vi "Configure.vi"(0 "session in":T6[](array[typedef]) {"rx baseband session"."3630 session"."Address Space" items=["VXI/VME A16"=1, "VXI/VME A24"=2, "VXI/VME A32"=3, "VXI/VME A64"=4, "PXI Memory Allocations"=9, "PXI Configuration"=10, "PXI BAR0"=11, "PXI BAR1"=12, "PXI BAR2"=13, "PXI BAR3"=14, "PXI BAR4"=15, "PXI BAR5"=16]; "tx baseband session"."3610 session"."Address Space" items=["VXI/VME A16"=1, "VXI/VME A24"=2, "VXI/VME A32"=3, "VXI/VME A64"=4, "PXI Memory Allocations"=9, "PXI Configuration"=10, "PXI BAR0"=11, "PXI BAR1"=12, "PXI BAR2"=13, "PXI BAR3"=14, "PXI BAR4"=15, "PXI BAR5"=16]}, 7 "device configuration [channel]":T3[](array[typedef])=[{"port select"=enum."Loopback", "Rx hardware configuration"={"gain (dB)"=15.0, "frequency (Hz)"=12000000000.0, "mmWave adapter"="None", "adapter active port"=""}, "Tx hardware configuration"={"gain (dB)"=-15.0, "frequency (Hz)"=12000000000.0, "mmWave adapter"="None", "adapter active port"=""}}] {"Tx hardware configuration"."frequency (Hz)" format="%#_6p"; "Rx hardware configuration"."frequency (Hz)" format="%#_6p"}, 11 "error in":errorcluster, 12 "LO sources":T2={"RX/LO1 src"="Internal", "TX/LO1 src"="Internal", "LO2 src"="Internal"}, 13 "LO Export":T1) -> (4 "session out":T6[](array[typedef]) {"rx baseband session"."3630 session"."Address Space" items=["VXI/VME A16"=1, "VXI/VME A24"=2, "VXI/VME A32"=3, "VXI/VME A64"=4, "PXI Memory Allocations"=9, "PXI Configuration"=10, "PXI BAR0"=11, "PXI BAR1"=12, "PXI BAR2"=13, "PXI BAR3"=14, "PXI BAR4"=15, "PXI BAR5"=16]; "tx baseband session"."3610 session"."Address Space" items=["VXI/VME A16"=1, "VXI/VME A24"=2, "VXI/VME A32"=3, "VXI/VME A64"=4, "PXI Memory Allocations"=9, "PXI Configuration"=10, "PXI BAR0"=11, "PXI BAR1"=12, "PXI BAR2"=13, "PXI BAR3"=14, "PXI BAR4"=15, "PXI BAR5"=16]}, 8 "coerced device configuration [channel]":T3[](array[typedef])=[{"port select"=enum."Loopback", "Rx hardware configuration"={"gain (dB)"=15.0, "frequency (Hz)"=12000000000.0, "mmWave adapter"="None", "adapter active port"=""}, "Tx hardware configuration"={"gain (dB)"=-15.0, "frequency (Hz)"=12000000000.0, "mmWave adapter"="None", "adapter active port"=""}}] {"Tx hardware configuration"."frequency (Hz)" format="%#_6p"; "Rx hardware configuration"."frequency (Hz)" format="%#_6p"}, 15 "error out":errorcluster)   [LabVIEW 2019, in "mmWave HW Control.lvlib"]
uses:
  mmWave HW Control.lvlib
  Low-level/TypeDefs/Front End Configuration.ctl
  Low-level/TypeDefs/Channel Configuration.ctl
  <instrlib>/niMmWave/ni3620/Config/v1/Host/Public/Typedefs/mmWave Port.ctl
  Low-level/TypeDefs/Session.ctl
  <instrlib>/niMmWave/ni3620/Config/v1/Host/Public/High-Level/niMmWave Session.ctl
  <instrlib>/_niInstr/Register Bus/v0/Host/Public/Register Bus Session.ctl
  <instrlib>/_niInstr/Register Bus/v0/Host/Private/Session Data.ctl
  <instrlib>/niMmWave/ni3620/Config/v1/Host/Public/Typedefs/Board Information.ctl
  <instrlib>/niMmWave/ni3620/Config/v1/Host/Public/Typedefs/Hardware Revision.ctl
  <instrlib>/niMmWave/ni3620/Config/v1/Host/Public/Typedefs/Gain Mapping.ctl
  <instrlib>/niMmWave/ni3620/Config/v1/Host/Public/Typedefs/Correction Data.ctl
  <instrlib>/niMmWave/ni3620/Config/v1/Host/Public/Typedefs/Opera Characterization.ctl
  <instrlib>/niMmWave/ni3620/Config/v1/Host/Public/Corrections/Typedefs/Opera Characterization Main Header.ctl
  <instrlib>/niMmWave/ni3620/Config/v1/Host/Public/Corrections/Typedefs/Opera IF Board Information.ctl
  <instrlib>/niMmWave/ni3620/Config/v1/Host/Public/Corrections/Typedefs/Opera Characterization Instance Header.ctl
  <instrlib>/niMmWave/ni3620/Config/v1/Host/Public/Corrections/Typedefs/Opera Characterization Device Data Header.ctl
  <instrlib>/niMmWave/ni3620/Config/v1/Host/Public/Corrections/Typedefs/Opera LO Characterization Data Header.ctl
  <instrlib>/niMmWave/ni3620/Config/v1/Host/Public/Corrections/Typedefs/Opera IF Board Characterization Data Header.ctl
  <instrlib>/niMmWave/ni3620/Config/v1/Host/Public/Corrections/Typedefs/Opera Characterization Device Data.ctl
  <instrlib>/niMmWave/ni3620/Config/v1/Host/Public/Corrections/Typedefs/Opera LO2 Board Characterization Data.ctl
  <instrlib>/niMmWave/ni3620/Config/v1/Host/Public/Corrections/Typedefs/Opera LO Characterization Data.ctl
  <instrlib>/niMmWave/ni3620/Config/v1/Host/Public/Corrections/Typedefs/Opera IF Board Characterization Data.ctl
  <instrlib>/niMmWave/ni3620/Config/v1/Host/Public/Corrections/Typedefs/Opera IQ Impairment Data.ctl
  <instrlib>/niMmWave/ni3620/Config/v1/Host/Public/Typedefs/mmWave Adapter Session Data.ctl
  <instrlib>/niMmWave/ni3620/Config/v1/Host/Public/Typedefs/mmWave Adapter Data.ctl
  <instrlib>/niMmWave/ni3620/Config/v1/Host/Public/Typedefs/mmWave Adapter 2.ctl
  <instrlib>/niMmWave/ni3620/Config/v1/Shared/Typedefs/Subsystem ID.ctl
  <instrlib>/niMmWave/ni3620/Config/v1/Host/Public/Typedefs/mmWave Adapter Channel Information.ctl
  <instrlib>/niMmWave/ni3620/Config/v1/Host/Public/Typedefs/Temperature Coefficients.ctl
  <instrlib>/niMmWave/ni3620/Config/v1/Host/Public/Typedefs/mmWave Characterization.ctl
  <instrlib>/niMmWave/ni3620/Config/v1/Host/Public/Corrections/Typedefs/mmWave Characterization Main Header.ctl
  <instrlib>/niMmWave/ni3620/Config/v1/Host/Public/Corrections/Typedefs/mmWave Characterization Instance Header.ctl
  <instrlib>/niMmWave/ni3620/Config/v1/Host/Public/Typedefs/Session Cache.ctl
  <instrlib>/niMmWave/ni3620/Config/v1/Host/Public/Typedefs/LO2 settings cache.ctl
  <instrlib>/niMmWave/ni3620/Config/v1/Host/Public/Typedefs/LO2 source.ctl
  <instrlib>/niMmWave/ni3620/Config/v1/Host/Public/Typedefs/Desired and Coerced.ctl
  <instrlib>/niMmWave/ni3620/Config/v1/Host/Public/Typedefs/Export cache.ctl
  <instrlib>/niMmWave/ni3620/Config/v1/Host/Public/Typedefs/Path cache.ctl
  <instrlib>/niMmWave/ni3620/Config/v1/Host/Public/Typedefs/Daughterboard Type.ctl
  <instrlib>/niMmWave/ni3620/Config/v1/Host/Public/Typedefs/LO1 settings cache.ctl
  <instrlib>/niMmWave/ni3620/Config/v1/Host/Public/Typedefs/LO1 Source.ctl
  <instrlib>/niMmWave/ni3620/Config/v1/Host/Public/Typedefs/mmWave export cache.ctl
  <instrlib>/niMmWave/ni3620/Config/v1/Host/Private/Board/LO2/LO2 Board Configuration Cache.ctl
  <instrlib>/niMmWave/ni3620/Config/v1/Host/Public/Typedefs/reference clock routing settings.ctl
  <instrlib>/niMmWave/ni3620/Config/v1/Host/Public/Typedefs/LO2 routing settings.ctl
  <instrlib>/niMmWave/ni3620/Config/v1/Host/Private/Board/LO1/LO1 Board Configuration Cache.ctl
  <instrlib>/niMmWave/ni3620/Config/v1/Host/Public/Typedefs/LO1 source settings.ctl
  <instrlib>/niMmWave/ni3620/Config/v1/Host/Public/Typedefs/LO1 export settings.ctl
  <instrlib>/niMmWave/ni3620/Config/v1/Host/Public/Typedefs/LO1 mmWave settings.ctl
  Low-level/TypeDefs/Tx Baseband Session.ctl
  <instrlib>/niMmWave/ni3610 and ni3630/controls/public/Main Settings.ctl
  <vilib>/Instr/_visa.llb/VISA Register Access Address Space.ctl
  <instrlib>/niMmWave/ni3610 and ni3630/controls/public/Register Adresses.ctl
  <instrlib>/niMmWave/ni3610 and ni3630/controls/public/Base Card Type.ctl
  <instrlib>/niMmWave/ni3610 and ni3630/controls/private/IQ Card Revision.ctl
  <instrlib>/niMmWave/ni3610 and ni3630/controls/public/Board Capability.ctl
  Low-level/TypeDefs/Blank FPGA Reference.ctl
  Low-level/TypeDefs/Rx Baseband Session.ctl
  Low-level/TypeDefs/Hardware Configuration.ctl
  Low-level/TypeDefs/Direction.ctl
  Low-level/TypeDefs/Gain Ranging.ctl
  Low-level/TypeDefs/PXI Trigger Bus Info.ctl
  LO sources.ctl
  LO export.ctl
  <instrlib>/niMmWave/ni3620/Config/v1/Host/Public/Typedefs/Rx IF signal source.ctl
  <instrlib>/niMmWave/ni3620/Config/v1/Host/Public/Typedefs/Tx IF signal destination.ctl
  <instrlib>/niMmWave/ni3620/Config/v1/Host/niMmWave Config v1 Host.lvlib
  <instrlib>/niMmWave/ni3610 and ni3630/ni3610_and_ni3630_Driver_Lib.lvlib
  <instrlib>/_niInstr/Register Bus/v0/Host/niInstr Register Bus v0 Host.lvlib
  <instrlib>/niMmWave/ni3620/Config/v1/Shared/niMmWave Config v1 Shared.lvlib
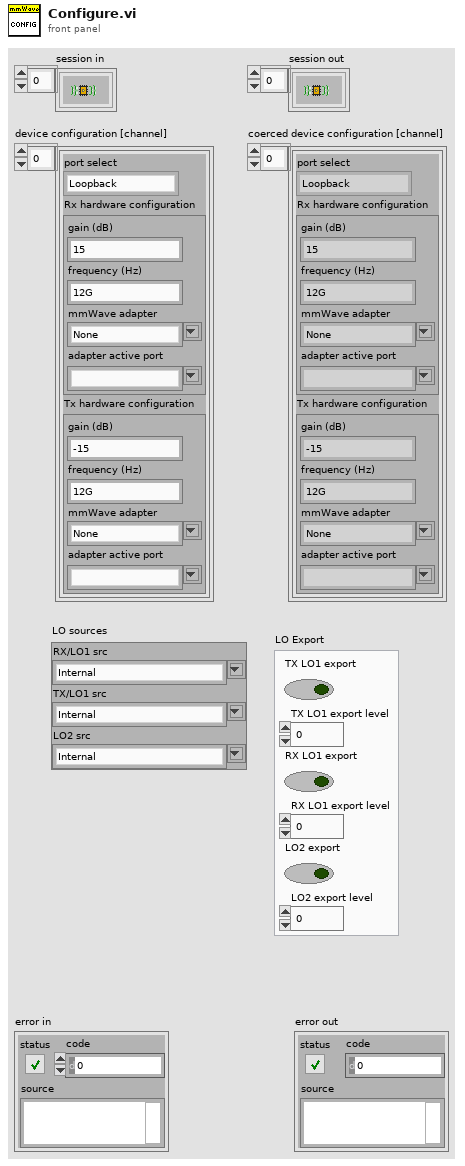
[diagram p1: front panel]
types:
  T1 = typedef "mmWave HW Control.lvlib/LO export.ctl" = cluster{"TX LO1 export":bool, "TX LO1 export level":dbl, "RX LO1 export":bool, "RX LO1 export level":dbl, "LO2 export":bool, "LO2 export level":dbl}
  T2 = typedef "mmWave HW Control.lvlib/LO sources.ctl" = cluster{"RX/LO1 src":string, "TX/LO1 src":string, "LO2 src":string}
  T3 = typedef "Front End Configuration.ctl" = cluster{"port select":enum16{"IF Port", "Loopback", "Sync Port"}, "Rx hardware configuration":T4, "Tx hardware configuration":T4}
  T4 = typedef "Channel Configuration.ctl" = cluster{"gain (dB)":dbl, "frequency (Hz)":dbl, "mmWave adapter":string, "adapter active port":T5}
  T5 = typedef "niMmWave Config v1 Host.lvlib/mmWave Port.ctl" = string
  T6 = typedef "Session.ctl" = cluster{"3620 session":refnum<queue>, "tx baseband session":T7, "rx baseband session":T15, "tx gain (dB)":dbl, "rx gain (dB)":dbl, "hardware configuration":T16, "gain ranging":T18[], "pxi trigger bus information":T19}
  T7 = typedef "Tx Baseband Session.ctl" = cluster{"3610 session":T8, "7902 reference":T14}
  T8 = typedef "ni3610_and_ni3630_Driver_Lib.lvlib/Main Settings.ctl" = cluster{"VISA resource name":refnum<visa-resource-name>, "Address Space":T9, "window_offset":u32, "register_addresses":T10, "required_MM_fpga_version":cluster{"signature":u32, "hardware":u32, "current revision":u32, "oldest revision":u32}, "CPLD Oldest Compat Version ":cluster{"hardware":u32, "CPLD firmware":u32}, "MM_FPGA_image_location":string, "is_init":bool, "card_type":T11, "DacLmkConfigFileName":string, "AdcLmkConfigFileName":string, "AdcConfigFileName":string, "DacConfigFileName_RevA":string, "DacConfigFileName_RevB":string, "Mulde hardware revision":u8, "bypass DAC PLL\n":bool, "IQ Card Revision":T12, "board capability":T13}
  T9 = typedef "VISA Register Access Address Space.ctl" = u16
  T10 = typedef "ni3610_and_ni3630_Driver_Lib.lvlib/Register Adresses.ctl" = cluster{"MM based Registers":cluster{"Revision":u32, "OldestCompatRev":u32, "signature":u32, "scratch":u32, "LedControl":u32, "BoardHwRev":u32, "BoardControl":u32, "ThermalStatus":u32, "BasebandStatus":u32, "BasebandControl":u32, "BasebandAuxSetup":u32, "BasebandAuxStatus":u32, "LmkSyncOutSetup":u32, " AdcSyncOutSetup":u32, " InjSyncOutSetup":u32, " PxiTrig0OutSetup":u32, " PxiTrig1OutSetup":u32, " PxiTrig2OutSetup":u32, " PxiTrig3OutSetup":u32, " PxiTrig4OutSetup":u32, " PxiTrig5OutSetup":u32, " PxiTrig6OutSetup":u32, " PxiTrig7OutSetup":u32}, "CPLD based Registers":cluster{"SlaveSignature":u32, "SlaveRevision":u32, "SlaveOldestCompatRev":u32, "SlaveScratch":u32, "SlaveSetup":u32, "SlaveStatus":u32, "IDacReg_offset":u32, "LMKRegGrp0_offset":u32, "QDacReg_offset":u32, "BrdTempSensorVal":u32, "TempSensorPowerDown":u32, "GPIOReg_offset":u32, "IAdcReg_offset":u32, "QAdcReg_offset":u32, "LMKRegGrp1_offset":u32, "QadcTempSensorVal":u32, "IadcTempSensorVal":u32, "RevisionReg":u32, "VcxoReg":u32, "CpldStatusReg":u32, "PowerReg":u32, "VBiasEnReg":u32, "ExtRefOeReg":u32, "QdacCtrlReg":u32, "QdacStatusReg":u32, "IdacCtrlReg":u32, "IdacStatusReg":u32, "QdacJtagIn":u32, "QdacJtagOut":u32, "IdacJtagIn":u32, "IdacJtagOut":u32, "IqDcSetupReg":u32, "QadcStatusReg":u32, "IadcStatusReg":u32, "BrdSetupReg":u32, "IqDcRevisionReg":u32, "PllStatusReg":u32, "EndpointScratchReg":u32, "AdcSyncCfgReg":u32, "IqCardOpampReg":u32}, "CPLD Register Offset":u32, "MM  Register Offset":u32, " PxiTrig0OutSetup":u32}
  T11 = typedef "ni3610_and_ni3630_Driver_Lib.lvlib/Base Card Type.ctl" = enum16{"unspecified", "ADC", "DAC"}
  T12 = typedef "ni3610_and_ni3630_Driver_Lib.lvlib/IQ Card Revision.ctl" = enum16{"RevA", "RevB", "RevC", "RevD"}
  T13 = typedef "ni3610_and_ni3630_Driver_Lib.lvlib/Board Capability.ctl" = cluster{"baseband sync":enum16{"no baseband sync", "baseband sync"}}
  T14 = typedef "Blank FPGA Reference.ctl" = refnum<k20>
  T15 = typedef "Rx Baseband Session.ctl" = cluster{"3630 session":T8, "7902 reference":T14}
  T16 = typedef "Hardware Configuration.ctl" = cluster{"direction":T17, "baseband only":bool}
  T17 = typedef "Direction.ctl" = enum16{"Transceiver", "Receiver", "Transmitter"}
  T18 = typedef "Gain Ranging.ctl" = cluster{"gain ranging active scope":string, "gain ranging stream session":refnum<k20>}
  T19 = typedef "PXI Trigger Bus Info.ctl" = cluster{"chassis resource name":refnum<visa-resource-name>, "7902R (TX)":i16, "3610 (TX)":i16, "3620 (IF)":i16, "3630 (RX)":i16, "7902R (RX)":i16}
  T20 = typedef "niMmWave Config v1 Host.lvlib/Tx IF signal destination.ctl" = enum16{"IF Output", "IF Loopback", "Cal Output", "Disabled"}
  T21 = typedef "niMmWave Config v1 Host.lvlib/Rx IF signal source.ctl" = enum16{"IF Input", "IF Loopback", "External Cal Input", "Internal Cal Input"}
  T22 = typedef "niMmWave Config v1 Host.lvlib/Opera IQ Impairment Data.ctl" = cluster{"Gain Imbalance (linear)":dbl, "Phase Offset (radians)":dbl, "Offset ":cdb}
  T23 = typedef "niMmWave Config v1 Host.lvlib/IQ Inversion.ctl" = cluster{"invert i":bool, "invert q":bool}
  T24 = typedef "niMmWave Config v1 Host.lvlib/niMmWave Session.ctl" = cluster{"register bus ":T25, "board information":T26, "IF gain tables":cluster{"Gain Table":T28[]}[], "IF channel correction data":T29[], "ni3620 characterization data":T30, "mmWave adapter session data":T41, "session cache":T50, "lo2 board configuration cache":T60, "lo1 rx board configuration cache":T63, "lo1 tx board configuration cache":T63}
  T25 = typedef "niInstr Register Bus v0 Host.lvlib/Register Bus Session.ctl" = refnum<queue>
  T26 = typedef "niMmWave Config v1 Host.lvlib/Board Information.ctl" = cluster{"product code":u16, "hardware revision":T27, "serial number":u64}
  T27 = typedef "niMmWave Config v1 Host.lvlib/Hardware Revision.ctl" = enum16{"Unknown", "A", "B", "C", "D", "E", "F", "G", "H", "I", "J"}
  T28 = typedef "niMmWave Config v1 Host.lvlib/Gain Mapping.ctl" = cluster{"Gain":dbl, "Gain Settings":variant[]}
  T29 = typedef "niMmWave Config v1 Host.lvlib/Correction Data.ctl" = cluster{"Frequencies (Hz)":dbl[], "Nominal Gain Values (dB)":dbl[], "Measured Gain Values (dB)":dbl[][]}
  T30 = typedef "niMmWave Config v1 Host.lvlib/Opera Characterization.ctl" = cluster{"Characterization Data Valid?":bool, "ni3620 characterization main header":T31, "ni3620 characterization instance header":T33, "ni3620 characterization device data header":T34, "ni3620 characterization device data":T37}
  T31 = typedef "niMmWave Config v1 Host.lvlib/Opera Characterization Main Header.ctl" = cluster{"Header Checksum":u32, "Product Code":u16, "Module Serial Number":u64, "Hardware Current Version":u16, "Hardware Oldest Compatible Version":u16, "EEPROM Map Current Version":u16, "EEPROM Map Oldest Compatible Version":u16, "User Password":string, "Factory Characterization Header Address":u32, "User Characterization Header Address":u32, "Recommended Correction Interval (months)":u16, "Mighty Mouse Hardware Current Version":u16, "Mighty Mouse Serial Number":u64, "LO2 Board Hardware Current Version":u16, "LO2 Board Serial Number":u64, "Number of IF Boards":u8, "IF Boards":T32[], "Future Growth":u16}
  T32 = typedef "niMmWave Config v1 Host.lvlib/Opera IF Board Information.ctl" = cluster{"IF Board ID":u16, "IF Board Hardware Current Version":u16, "IF Board Serial Number":u64}
  T33 = typedef "niMmWave Config v1 Host.lvlib/Opera Characterization Instance Header.ctl" = cluster{"Header Checksum":u32, "Characterization Date":timestamp, "Characterization Temperature (C)":dbl, "Miscellaneous Information":string, "Device Characterization Header Address":u32, "Future Growth":u16}
  T34 = typedef "niMmWave Config v1 Host.lvlib/Opera Characterization Device Data Header.ctl" = cluster{"Header Checksum":u32, "Number of LO2 Export Paths":u8, "LO2 Export Paths":T35[], "Number of IF Boards":u8, "IF Boards":T36[], "Characterization Data Address":u32, "Future Growth":u16}
  T35 = typedef "niMmWave Config v1 Host.lvlib/Opera LO Characterization Data Header.ctl" = cluster{"LO Path Number of Frequencies":u16, "LO Path Number of Gain Values":u16}
  T36 = typedef "niMmWave Config v1 Host.lvlib/Opera IF Board Characterization Data Header.ctl" = cluster{"Number of LO1 Export Paths":u8, "LO1 Export Paths":T35[], "IF Path Number of Gain Frequencies":u16, "IF Path Number of Gain Stages":u16, "IF Path Gain Stages Number of Gain Values":u16[], "IF Path Number of IQ Impairment Frequencies":u16}
  T37 = typedef "niMmWave Config v1 Host.lvlib/Opera Characterization Device Data.ctl" = cluster{"LO2 Board Characterization Data":T38, "IF Board Characterization Data":T40[]}
  T38 = typedef "niMmWave Config v1 Host.lvlib/Opera LO2 Board Characterization Data.ctl" = cluster{"Data Checksum":u32, "TXCO Reference DAC Value":u16, "LO2 Export Paths":T39[]}
  T39 = typedef "niMmWave Config v1 Host.lvlib/Opera LO Characterization Data.ctl" = cluster{"Frequencies":dbl[], "Gain Values":dbl[], "Measured Gain / Power Values":dbl[][]}
  T40 = typedef "niMmWave Config v1 Host.lvlib/Opera IF Board Characterization Data.ctl" = cluster{"Data Checksum":u32, "LO1 Export Paths":T39[], "IF Path Gain Frequencies":dbl[], "IF Path Gain Stages Gain Values":cluster{"Gain Values":dbl[]}[], "Measured Maximum Gain (dB)":dbl[], "IF Path Gain Stages Measured Gain Values (dB)":cluster{"Measured Gain Values (dB)":dbl[][]}[], "IF Path IQ Impairment Frequencies":dbl[], "Measured IQ Impairments":T22[]}
  T41 = typedef "niMmWave Config v1 Host.lvlib/mmWave Adapter Session Data.ctl" = cluster{"mmWave0 chain size":u8, "mmWave1 chain size ":u8, "mmWave adapters":T42[]}
  T42 = typedef "niMmWave Config v1 Host.lvlib/mmWave Adapter Data.ctl" = cluster{"scope":string, "mmWave Adapter type":T43, "board information":T26, "subsystem":T44, "serial address":u8, "channels":T45[], "channel gain tables":cluster{"Gain Table":T28[]}[], "channel correction data":T29[], "channel temperature coefficients":T46[], "characterization data":T47, "board configuration cache":variant}
  T43 = typedef "niMmWave Config v1 Host.lvlib/mmWave Adapter 2.ctl" = enum16{"None", "NI 3647 71-76 GHz", "NI 3657 71-76 GHz", "NI 5580 55-68 GHz", "NI 5580 55-68 GHz Prototype Deck", "NI 3602 27.5-29.5 GHz", "NI 3642 27.5-29.5 GHz", "NI 3652 27.5-29.5 GHz", "NI 3603 37.0-43.5 GHz", "NI 3643 37.0-43.5 GHz", "NI 3653 37.0-43.5 GHz", "NI 3602 24.25-33.40 GHz", "NI 3642 24.25-33.40 GHz", "NI 3652 24.25-33.40 GHz"}
  T44 = typedef "niMmWave Config v1 Shared.lvlib/Subsystem ID.ctl" = enum8{"Identification", "Board Config", "Rx LO1", "Tx LO1", "LO2", "mmWave0", "mmWave1", "Rx LO1 Core", "Tx LO1 Core", "LO2 Core", "mmWave0 Core", "mmWave1 Core", "Gain Ranging", "mmWave mapping"}
  T45 = typedef "niMmWave Config v1 Host.lvlib/mmWave Adapter Channel Information.ctl" = cluster{"channel":string, "supported ports":string[], "active port":string}
  T46 = typedef "niMmWave Config v1 Host.lvlib/Temperature Coefficients.ctl" = cluster{"frequencies (Hz)":dbl[], "gains (dB)":dbl[], "temp coefficients [gain][freq]":dbl[][]}
  T47 = typedef "niMmWave Config v1 Host.lvlib/mmWave Characterization.ctl" = cluster{"Characterization Data Valid?":bool, "mmWave Characterization Main Header":T48, "mmWave Characterization Instance Header":T49, "mmWave Characterization Device Data Header":variant, "mmWave Characterization Device Data":variant}
  T48 = typedef "niMmWave Config v1 Host.lvlib/mmWave Characterization Main Header.ctl" = cluster{"Header Checksum":u32, "Product Code":u16, "Serial Number":u64, "Hardware Current Version":u16, "Hardware Oldest Compatible Version":u16, "EEPROM Map Current Version":u16, "EEPROM Map Oldest Compatible Version":u16, "Hardware Capabilities":u8, "User Password":string, "Factory Characterization Header Address":u32, "User Characterization Header Address":u32, "Recommended Correction Interval (months)":u16, "Future Growth":u16}
  T49 = typedef "niMmWave Config v1 Host.lvlib/mmWave Characterization Instance Header.ctl" = cluster{"Header Checksum":u32, "Characterization Date":timestamp, "Characterization Temperature (C)":dbl, "Miscellaneous Information":string, "Device Characterization Header Address":u32, "Future Growth":u16}
  T50 = typedef "niMmWave Config v1 Host.lvlib/Session Cache.ctl" = cluster{"Gain Corrections Enabled":bool, "LO2 Settings":T51, "TxRx Path Settings":T55[], "LO Corrections Enabled":bool}
  T51 = typedef "niMmWave Config v1 Host.lvlib/LO2 settings cache.ctl" = cluster{"Source":T52, "Frequency":T53, "Export Settings":T54}
  T52 = typedef "niMmWave Config v1 Host.lvlib/LO2 source.ctl" = enum16{"Internal", "LO2_IN"}
  T53 = typedef "niMmWave Config v1 Host.lvlib/Desired and Coerced.ctl" = cluster{"Desired":dbl, "Coerced":dbl}
  T54 = typedef "niMmWave Config v1 Host.lvlib/Export cache.ctl" = cluster{"Export Enabled":bool, "Path Gain":T53}
  T55 = typedef "niMmWave Config v1 Host.lvlib/Path cache.ctl" = cluster{"Daughterboard":T56, "current mmWave Adapter":T43, "current mmWave adapter index":i32, "Channel Enabled":bool, "Gain":T53, "Frequency":T53, "LO1":T57, "IF Route":variant}
  T56 = typedef "niMmWave Config v1 Host.lvlib/Daughterboard Type.ctl" = enum16{"3620 RX", "3620 TX"}
  T57 = typedef "niMmWave Config v1 Host.lvlib/LO1 settings cache.ctl" = cluster{"Source":T58, "Frequency":T53, "LO1 mmWave":T59, "LO1 Export":T54}
  T58 = typedef "niMmWave Config v1 Host.lvlib/LO1 Source.ctl" = enum16{"Internal", "LO1_IN"}
  T59 = typedef "niMmWave Config v1 Host.lvlib/mmWave export cache.ctl" = cluster{"Export Settings":T54, "AGC Enabled":bool, "Doubler Enabled":bool}
  T60 = typedef "niMmWave Config v1 Host.lvlib/LO2 Board Configuration Cache.ctl" = cluster{"reference clock routing settings":T61, "LO2 routing settings":T62}
  T61 = typedef "niMmWave Config v1 Host.lvlib/reference clock routing settings.ctl" = cluster{"reference clock source":enum16{"PXI_Clk10", "Ref In"}, "export reference clock ":bool}
  T62 = typedef "niMmWave Config v1 Host.lvlib/LO2 routing settings.ctl" = cluster{"LO2 Source":T52, "export LO2":bool, "LO2 output attenuation":fxp<+,7,5>}
  T63 = typedef "niMmWave Config v1 Host.lvlib/LO1 Board Configuration Cache.ctl" = cluster{"LO1 source routing settings":T64, "LO1 export routing settings":T65, "LO1 mmWave routing settings":T66}
  T64 = typedef "niMmWave Config v1 Host.lvlib/LO1 source settings.ctl" = cluster{"LO1 source":T58, "LO1 source attenuation":fxp<+,7,5>}
  T65 = typedef "niMmWave Config v1 Host.lvlib/LO1 export settings.ctl" = cluster{"export LO1":bool, "LO1 export attenuation":fxp<+,7,5>}
  T66 = typedef "niMmWave Config v1 Host.lvlib/LO1 mmWave settings.ctl" = cluster{"LO1 mmWave route":enum16{"Chop Cal", "Doubler", "Bypass"}, "LO1 mmWave attenuation":fxp<+,5,5>}
  T67 = typedef "ni3610_and_ni3630_Driver_Lib.lvlib/Baseband IQ Characterization Device Data.ctl" = cluster{"Checksum":u32, "Channel Delay":dbl, "Imbalance":cluster{"Gain Imbalance":dbl, "Phase Imbalance":dbl}, "DC Offset":cluster{"I DC Offset":dbl, "Q DC Offset":dbl}}
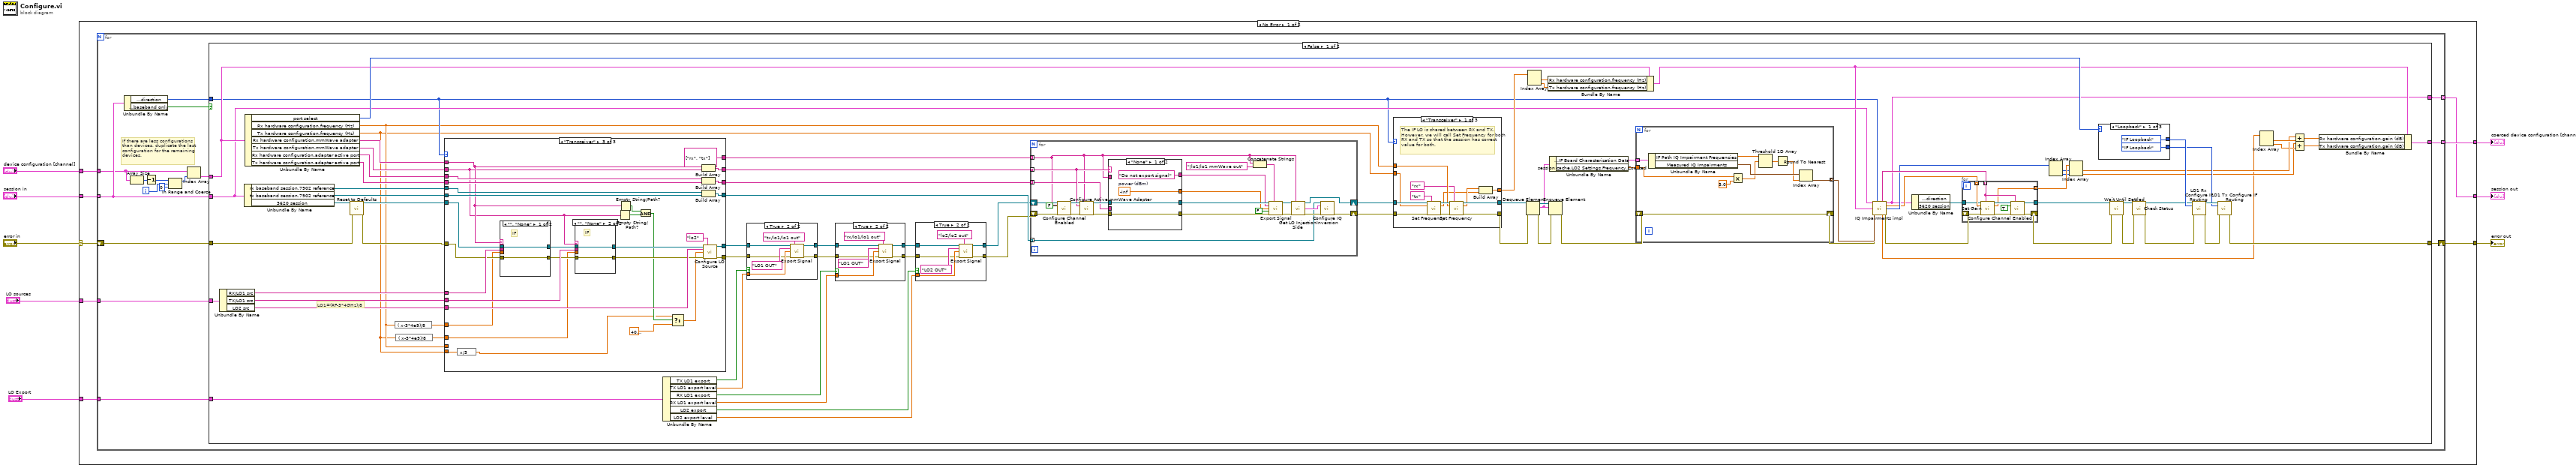
[diagram p0: block diagram]
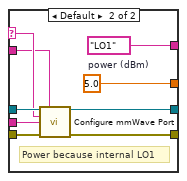
[diagram p5: hidden frame]
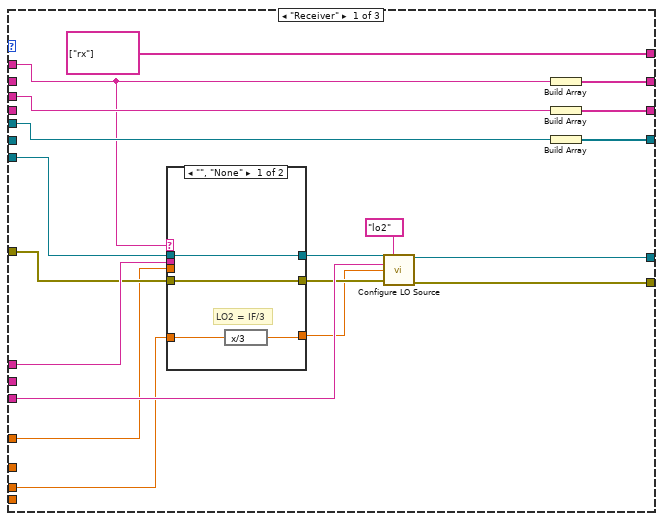
[diagram p6: hidden frame]
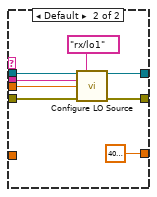
[diagram p7: hidden frame]
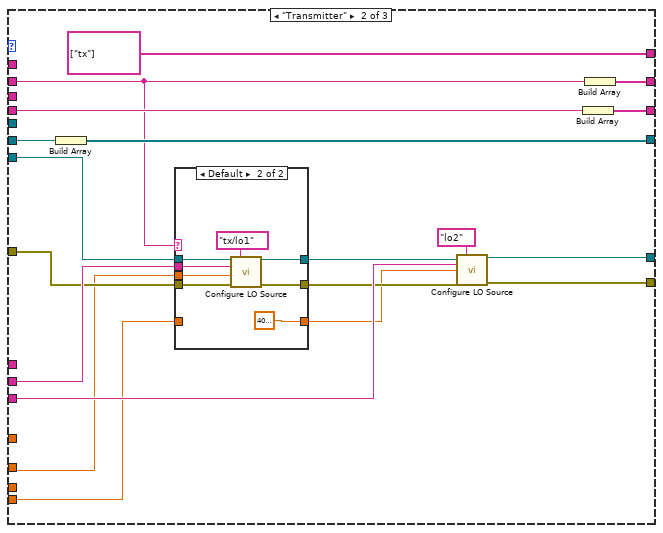
[diagram p8: hidden frame]
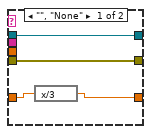
[diagram p9: hidden frame]
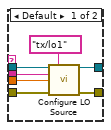
[diagram p10: hidden frame]
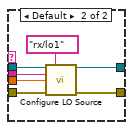
[diagram p11: hidden frame]
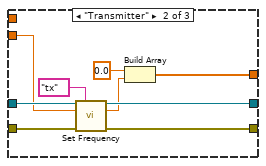
[diagram p12: hidden frame]
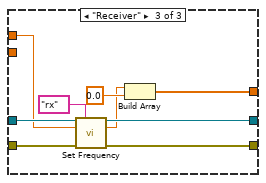
[diagram p13: hidden frame]
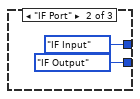
[diagram p14: hidden frame]
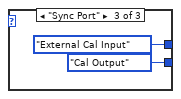
[diagram p15: hidden frame]
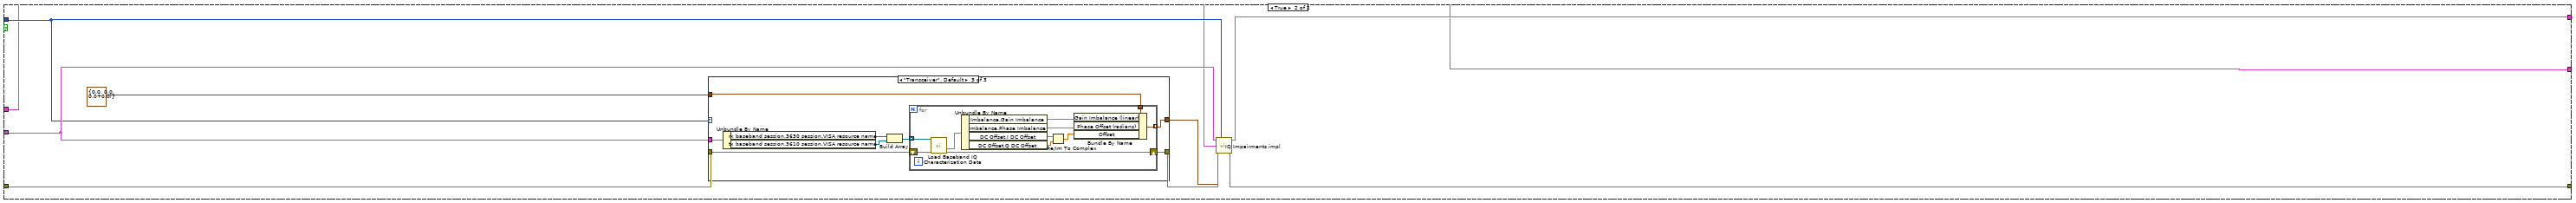
[diagram p16: hidden frame]
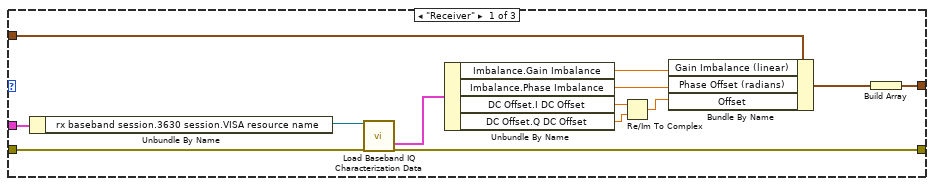
[diagram p17: hidden frame]
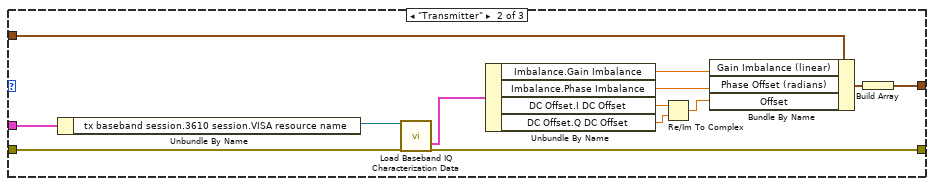
[diagram p18: hidden frame]
diagram:
  n1 = case shown="No Error" "error in" {
    selector: "error in" -> [w16 w405]
    tunnel: "device configuration [channel]" -> [w11 _]
    tunnel: "session in" -> [w12 w404]
    tunnel: [w15 w405] -> w7
    tunnel: [w14 _] -> w6
    tunnel: [w13 w404] -> w5
    tunnel: "LO sources" -> [w10 _]
    tunnel: "LO Export" -> [w9 _]
    frame No Error {
      n2 = for {
        shift-right: [w31] -> w15
        shift-left: w16 -> [w32]
        tunnel: w11 -> [w20]
        tunnel: [w30] -> w14 mode=indexing
        tunnel: w12 -> [w21] mode=indexing
        tunnel: [w29] -> w13 mode=indexing
        tunnel: w10 -> [w18]
        tunnel: w9 -> [w17]
        i -> [w22]
        # "If there are less configurations than devices, duplicate the last configuration for the remaining devices."
        n3 = Unbundle By Name(w21) -> ("hardware configuration.direction"=w28:T17, "hardware configuration.baseband only"=w27:bool)
        n4 = Array Size(array=w20) -> (size(s)=w25:i32)
        n5 = Decrement(x=w25) -> (x-1=w24:i32)
        n6 = In Range and Coerce(upper limit=w24, x=w22, lower limit=0) -> (coerced(x)=w23:i32)  [unwired: 1 out]
        n7 = Index Array(array=w20, index=w23) -> (element=w19:T3)
        n8 = case shown="False" w27 {
          tunnel: w19 -> [w86 w350]
          tunnel: w32 -> [w69 w358]
          tunnel: w21 -> [w68 w352]
          tunnel: [w93 w354] -> w31
          tunnel: w28 -> [w58 w351]
          tunnel: [w105 w350] -> w30
          tunnel: [w60 w353] -> w29
          tunnel: w18 -> [w57 _]
          tunnel: w17 -> [w49 _]
          frame False {
            # "LO1=(RF-3*4GHz)/8"
            n9 = Unbundle By Name(w57) -> ("RX/LO1 src"=w54:string, "TX/LO1 src"=w53:string, "LO2 src"=w52:string)
            n10 = Unbundle By Name(w68) -> ("rx baseband session.7902 reference"=w76:T14, "tx baseband session.7902 reference"=w75:T14, "3620 session"=w70:refnum<queue>)
            n11 = Unbundle By Name(w86) -> ("port select"=w109:enum16{"IF Port", "Loopback", "Sync Port"}, "Rx hardware configuration.frequency (Hz)"=w34:dbl, "Tx hardware configuration.frequency (Hz)"=w33:dbl, "Rx hardware configuration.mmWave adapter"=w80:string, "Tx hardware configuration.mmWave adapter"=w79:string, "Rx hardware configuration.adapter active port"=w73:T5, "Tx hardware configuration.adapter active port"=w71:T5)
            n12 = call <instrlib>:"Reset to Defaults.vi"("session in"=w70, "error in"=w69) -> ("session out"=w56:refnum<queue>, "error out"=w55:errorcluster)  [unwired: 12 in]
            n13 = expression code="( x-3*4e9)/8"(w34) -> (w51:dbl)
            n14 = expression code="( x-3*4e9)/8"(w33) -> (w50:dbl)
            n15 = case shown="\"Transceiver\"" w58 {
              tunnel: [string[] ["rx"] ("Array") string[] ["tx"] ("Array") string[] ["rx", "tx"] ("Array")] -> w82
              tunnel: [w199 w230 w273] -> w81
              tunnel: w80 -> [w184 _ w250]
              tunnel: w79 -> [_ w215 w248]
              tunnel: w76 -> [w198 _ w272]
              tunnel: w75 -> [_ w229 w270]
              tunnel: [w197 w228 w271] -> w74
              tunnel: w73 -> [w195 _ w269]
              tunnel: [w196 w227 w267] -> w72
              tunnel: w71 -> [_ w226 w268]
              tunnel: w56 -> [w194 w223 w263]
              tunnel: w55 -> [w188 w219 w258]
              tunnel: [w191 w222 w262] -> w47
              tunnel: w54 -> [w190 _ w261]
              tunnel: w53 -> [_ w220 w260]
              tunnel: w52 -> [w189 w221 w259]
              tunnel: [w186 w217 w255] -> w46
              tunnel: w51 -> [w185 _ w254]
              tunnel: w50 -> [_ w216 w253]
              tunnel: w34 -> [w182 _ _]
              tunnel: w33 -> [_ w213 w249]
              frame "Receiver" {
                n16 = case shown="\"\", \"None\"" w184 {
                  tunnel: w194 -> [w204 w212]
                  tunnel: [w204 w210] -> w193
                  tunnel: w190 -> [_ w209]
                  tunnel: w188 -> [w203 w208]
                  tunnel: [w203 w207] -> w187
                  tunnel: w185 -> [_ w206]
                  tunnel: [w201 4000000000.0 ("frequency (Hz)")] -> w183
                  tunnel: w182 -> [w202 _]
                  frame "", "None" {
                    # "LO2 = IF/3"
                    n17 = expression code="x/3"(w202) -> (w201:dbl)
                  }
                  frame Default {
                    n18 = call <instrlib>:"Configure LO Source.vi"("session in"=w212, "scope"="rx/lo1", "LO source"=w209, "frequency (Hz)"=w206, "error in"=w208) -> ("session out"=w210:refnum<queue>, "error out"=w207:errorcluster)  [unwired: 9 in]
                  }
                }
                n19 = call <instrlib>:"Configure LO Source.vi"("session in"=w193, "scope"="lo2", "LO source"=w189, "frequency (Hz)"=w183, "error in"=w187) -> ("session out"=w191:refnum<queue>, "error out"=w186:errorcluster)  [unwired: 9 in]
                n20 = Build Array(w184) -> (w199:string[])
                n21 = Build Array(w195) -> (w196:T5[])
                n22 = Build Array(w198) -> (w197:T14[])
              }
              frame "Transmitter" {
                n23 = Build Array(w229) -> (w228:T14[])
                n24 = case shown="Default" w215 {
                  tunnel: [w235 w242] -> w225
                  tunnel: w223 -> [w235 w241]
                  tunnel: w220 -> [_ w240]
                  tunnel: w219 -> [w234 w239]
                  tunnel: [w234 w238] -> w218
                  tunnel: w216 -> [_ w237]
                  tunnel: [w232 4000000000.0 ("frequency (Hz)")] -> w214
                  tunnel: w213 -> [w233 _]
                  frame "", "None" {
                    n25 = expression code="x/3"(w233) -> (w232:dbl)
                  }
                  frame Default {
                    n26 = call <instrlib>:"Configure LO Source.vi"("session in"=w241, "scope"="tx/lo1", "LO source"=w240, "frequency (Hz)"=w237, "error in"=w239) -> ("session out"=w242:refnum<queue>, "error out"=w238:errorcluster)  [unwired: 9 in]
                  }
                }
                n27 = call <instrlib>:"Configure LO Source.vi"("session in"=w225, "scope"="lo2", "LO source"=w221, "frequency (Hz)"=w214, "error in"=w218) -> ("session out"=w222:refnum<queue>, "error out"=w217:errorcluster)  [unwired: 9 in]
                n28 = Build Array(w226) -> (w227:T5[])
                n29 = Build Array(w215) -> (w230:string[])
              }
              frame "Transceiver" {
                n30 = expression code="x/3"(w249) -> (w246:dbl)
                n31 = case shown="\"\", \"None\"" w250 {
                  tunnel: [w285 w291] -> w266
                  tunnel: w263 -> [w285 w290]
                  tunnel: w261 -> [_ w289]
                  tunnel: w258 -> [w284 w288]
                  tunnel: [w284 w287] -> w257
                  tunnel: w254 -> [_ w286]
                  frame "", "None" {
                    # "IF"
                  }
                  frame Default {
                    n32 = call <instrlib>:"Configure LO Source.vi"("session in"=w290, "scope"="rx/lo1", "LO source"=w289, "frequency (Hz)"=w286, "error in"=w288) -> ("session out"=w291:refnum<queue>, "error out"=w287:errorcluster)  [unwired: 9 in]
                  }
                }
                n33 = case shown="\"\", \"None\"" w248 {
                  tunnel: w266 -> [w280 w283]
                  tunnel: [w279 w283] -> w265
                  tunnel: w260 -> [w278 _]
                  tunnel: w257 -> [w277 w282]
                  tunnel: [w276 w282] -> w256
                  tunnel: w253 -> [w275 _]
                  frame Default {
                    n34 = call <instrlib>:"Configure LO Source.vi"("session in"=w280, "scope"="tx/lo1", "LO source"=w278, "frequency (Hz)"=w275, "error in"=w277) -> ("session out"=w279:refnum<queue>, "error out"=w276:errorcluster)  [unwired: 9 in]
                  }
                  frame "", "None" {
                    # "IF"
                  }
                }
                n35 = Empty String/Path?(string/path=w248) -> (empty?=w252:bool)
                n36 = Empty String/Path?(string/path=w250) -> (empty?=w251:bool)
                n37 = And(x=w251, y=w252) -> (x .and. y?=w247:bool)
                n38 = Select(t=w246, s=w247, f=4000000000.0 ("frequency (Hz)")) -> (s? t:f=w244:dbl)
                n39 = Build Array(w250, w248) -> (w273:string[])
                n40 = Build Array(w269, w268) -> (w267:T5[])
                n41 = Build Array(w272, w270) -> (w271:T14[])
                n42 = call <instrlib>:"Configure LO Source.vi"("session in"=w265, "scope"="lo2", "LO source"=w259, "frequency (Hz)"=w244, "error in"=w256) -> ("session out"=w262:refnum<queue>, "error out"=w255:errorcluster)  [unwired: 9 in]
              }
            }
            n43 = Unbundle By Name(w49) -> ("TX LO1 export"=w48:bool, "TX LO1 export level"=w45:dbl, "RX LO1 export"=w43:bool, "RX LO1 export level"=w42:dbl, "LO2 export"=w40:bool, "LO2 export level"=w39:dbl)
            n44 = case shown="True" w48 {
              tunnel: w47 -> [w137 w141]
              tunnel: w46 -> [w136 w140]
              tunnel: w45 -> [_ w142]
              tunnel: [w137 w139] -> w44
              tunnel: [w136 w138] -> w38
              frame False {
              }
              frame True {
                n45 = call <instrlib>:"Export Signal.vi"("session in"=w141, "scope"="tx/lo1/lo1 out", "output terminal"="LO1 OUT", "gain / power (dB / dBm)"=w142, "error in"=w140) -> ("session out"=w139:refnum<queue>, "error out"=w138:errorcluster)  [unwired: 9 in]
              }
            }
            n46 = case shown="True" w43 {
              tunnel: w44 -> [w128 w132]
              tunnel: w42 -> [_ w133]
              tunnel: [w128 w131] -> w41
              tunnel: w38 -> [w127 w130]
              tunnel: [w127 w129] -> w37
              frame False {
              }
              frame True {
                n47 = call <instrlib>:"Export Signal.vi"("session in"=w132, "scope"="rx/lo1/lo1 out", "output terminal"="LO1 OUT", "gain / power (dB / dBm)"=w133, "error in"=w130) -> ("session out"=w131:refnum<queue>, "error out"=w129:errorcluster)  [unwired: 9 in]
              }
            }
            n48 = case shown="True" w40 {
              tunnel: w41 -> [w119 w123]
              tunnel: w39 -> [_ w124]
              tunnel: [w119 w122] -> w36
              tunnel: w37 -> [w118 w121]
              tunnel: [w118 w120] -> w35
              frame False {
              }
              frame True {
                n49 = call <instrlib>:"Export Signal.vi"("session in"=w123, "scope"="lo2/lo2 out", "output terminal"="LO2 OUT", "gain / power (dB / dBm)"=w124, "error in"=w121) -> ("session out"=w122:refnum<queue>, "error out"=w120:errorcluster)  [unwired: 9 in]
              }
            }
            n50 = for {
              tunnel: w82 -> [w149] mode=indexing
              shift-right: [w156] -> w78
              shift-left: w35 -> [w168]
              shift-right: [w163] -> w77
              shift-left: w36 -> [w167]
              tunnel: w81 -> [w160] mode=indexing
              tunnel: w74 -> [w155] mode=indexing
              tunnel: w72 -> [w159] mode=indexing
              n51 = call <instrlib>:"Configure Channel Enabled.vi"("session in"=w167, "scope"=w149, "enable channel?"=FALSE, "error in"=w168) -> ("session out"=w166:refnum<queue>, "error out"=w165:errorcluster)  [unwired: 10 in]
              n52 = call <instrlib>:"Configure Active mmWave Adapter.vi"("session in"=w166, "scope"=w149, "mmWave adapter"=w160, "error in"=w165) -> ("session out"=w161:refnum<queue>, "error out"=w162:errorcluster)  [unwired: 10 in]
              n53 = case shown="\"None\"" w160 {
                selector: w160 -> [_ w177]
                tunnel: w162 -> [w171 w181]
                tunnel: w161 -> [w172 w180]
                tunnel: [w172 w179] -> w152
                tunnel: [w171 w178] -> w154
                tunnel: w149 -> [_ w175]
                tunnel: w159 -> [_ w176]
                tunnel: ["Do not export signal" ("output terminal") "LO1" ("output terminal")] -> w147
                tunnel: [w169 w173] -> w146
                frame "None" {
                  w169 = -inf  # power (dBm)
                }
                frame Default {
                  w173 = 5.0  # power (dBm)
                  # "Power because internal LO1"
                  n54 = call <instrlib>:"Configure mmWave Port.vi"("session in"=w180, "scope"=w175, "mmWave adapter"=w177, "port"=w176, "error in"=w181) -> ("session out"=w179:refnum<queue>, "error out"=w178:errorcluster)  [unwired: 9 in]
                }
              }
              n55 = Concatenate Strings(w149, "/lo1/lo1 mmWave out" ("scope")) -> (w148:string)
              n56 = call <instrlib>:"Export Signal.vi"("session in"=w152, "scope"=w148, "output terminal"=w147, "gain / power (dB / dBm)"=w146, "enable AGC"=FALSE, "error in"=w154) -> ("session out"=w151:refnum<queue>, "error out"=w153:errorcluster)  [unwired: 8 in]
              n57 = call <instrlib>:"Get LO Injection Side.vi"("session in"=w151, "scope"=w149, "error in"=w153) -> ("session out"=w163:refnum<queue>, "IQ inversion"=w158:T23, "error out"=w157:errorcluster)  [unwired: 9 in, 1 out]
              n58 = call "Configure IQ Inversion.vi"("fpga reference in"=w155, "iq inversion"=w158, "error in"=w157) -> ("error out"=w156:errorcluster)  [unwired: 11 in, 1 out]
            }
            n59 = case shown="\"Transceiver\"" w58 {
              tunnel: w34 -> [w299 _ w315]
              tunnel: w33 -> [w294 w308 _]
              tunnel: w77 -> [w305 w314 w323]
              tunnel: w78 -> [w304 w313 w322]
              tunnel: [w295 w312 w321] -> w91
              tunnel: [w300 w311 w320] -> w90
              tunnel: [w303 w309 w318] -> w89
              frame "Transceiver" {
                # "The IF LO is shared between RX and TX.  However, we will call Set Frequency for both RX and TX so that the session has correct value for both."
                n60 = call <instrlib>:"Set Frequency.vi"("session in"=w305, "scope"="tx", "frequency (Hz)"=w294, "error in"=w304) -> ("session out"=w301:refnum<queue>, "coerced frequency (Hz)"=w293:dbl, "error out"=w297:errorcluster)  [unwired: 9 in]
                n61 = call <instrlib>:"Set Frequency.vi"("session in"=w301, "scope"="rx", "frequency (Hz)"=w299, "error in"=w297) -> ("session out"=w300:refnum<queue>, "coerced frequency (Hz)"=w296:dbl, "error out"=w295:errorcluster)  [unwired: 9 in]
                n62 = Build Array(w296, w293) -> (w303:dbl[])
              }
              frame "Transmitter" {
                n63 = call <instrlib>:"Set Frequency.vi"("session in"=w314, "scope"="tx", "frequency (Hz)"=w308, "error in"=w313) -> ("session out"=w311:refnum<queue>, "coerced frequency (Hz)"=w307:dbl, "error out"=w312:errorcluster)  [unwired: 9 in]
                n64 = Build Array(0.0 ("element"), w307) -> (w309:dbl[])
              }
              frame "Receiver" {
                n65 = call <instrlib>:"Set Frequency.vi"("session in"=w323, "scope"="rx", "frequency (Hz)"=w315, "error in"=w322) -> ("session out"=w320:refnum<queue>, "coerced frequency (Hz)"=w316:dbl, "error out"=w321:errorcluster)  [unwired: 9 in]
                n66 = Build Array(w316, 0.0 ("element")) -> (w318:dbl[])
              }
            }
            n67 = Dequeue Element(queue=w90, error in (no error)=w91) -> (queue out=w97:refnum<queue>, element=w94:T24, error out=w98:errorcluster)  [unwired: 1 in, 1 out]
            n68 = Index Array(array=w89) -> (element #1=w88:dbl, element #2=w87:dbl)  [unwired: 2 in]
            n69 = Bundle By Name(cluster=w86, "Rx hardware configuration.frequency (Hz)"=w88, "Tx hardware configuration.frequency (Hz)"=w87) -> (w67:T3)
            n70 = Enqueue Element(queue=w97, element=w94, error in (no error)=w98) -> (error out=w95:errorcluster)  [unwired: 1 in, 2 out]
            n71 = Unbundle By Name(w94) -> ("ni3620 characterization data.ni3620 characterization device data.IF Board Characterization Data"=w96:T40[], "session cache.LO2 Settings.Frequency.Coerced"=w92:dbl)
            n72 = for {
              tunnel: w96 -> [w333] mode=indexing
              shift-right: [w327] -> w65
              shift-left: w95 -> [w327]
              tunnel: [w328] -> w66 mode=indexing
              tunnel: w92 -> [w325]
              n73 = Unbundle By Name(w333) -> ("IF Path IQ Impairment Frequencies"=w331:dbl[], "Measured IQ Impairments"=w332:T22[])
              n74 = Multiply(x=w325, y=3.0) -> (x*y=w324:dbl)
              n75 = Threshold 1D Array(2:w324, 3:w331) -> (0:w330:dbl)  [unwired: 1 in]
              n76 = Round To Nearest(number=w330) -> (nearest integer value=w329:dbl)
              n77 = Index Array(array=w332, index=w329) -> (element=w328:T22)
            }
            n78 = call "IQ Impairments impl.vi"("session in"=w68, "direction"=w58, "device configuration"=w67, "IQ Impairments"=w66, "error in (no error)"=w65) -> ("scope"=w64:string[], "session out"=w60:T6, "configuration gain"=w61:dbl[], "Index"=w63:i32[], "gain (db)"=w59:dbl[], "error out"=w62:errorcluster)  [unwired: 5 in]
            n79 = Unbundle By Name(w60) -> ("3620 session"=w83:refnum<queue>)  [unwired: 1 out]
            n80 = for {
              tunnel: w83 -> [w334]
              shift-right: [w340] -> w117
              shift-left: w62 -> [w335]
              tunnel: [w339] -> w116
              tunnel: w64 -> [w338] mode=indexing
              tunnel: w61 -> [w337] mode=indexing
              tunnel: [w336] -> w101 mode=indexing
              n81 = call <instrlib>:"Set Gain.vi"("session in"=w334, "scope"=w338, "gain (dB)"=w337, "error in"=w335) -> ("session out"=w342:refnum<queue>, "coerced gain (dB)"=w336:dbl, "error out"=w343:errorcluster)  [unwired: 9 in]
              n82 = call <instrlib>:"Configure Channel Enabled.vi"("session in"=w342, "scope"=w338, "enable channel?"=TRUE, "error in"=w343) -> ("session out"=w339:refnum<queue>, "error out"=w340:errorcluster)  [unwired: 10 in]
            }
            n83 = Index Array(array=w63) -> (element #1=w100:i32, element #2=w99:i32)  [unwired: 2 in]
            n84 = Index Array(array=w101, index #1=w100, index #2=w99) -> (element #1=w107:dbl, element #2=w102:dbl)
            n85 = case shown="\"Loopback\"" w109 {
              tunnel: [Rx_IF_signal_source."IF Loopback" ("IF signal source") Rx_IF_signal_source."IF Input" ("IF signal source") Rx_IF_signal_source."External Cal Input" ("IF signal source")] -> w111
              tunnel: [Tx_IF_signal_destination."IF Loopback" ("IF signal destination") Tx_IF_signal_destination."IF Output" ("IF signal destination") Tx_IF_signal_destination."Cal Output" ("IF signal destination")] -> w110
              frame "Loopback" {
              }
              frame "IF Port" {
              }
              frame "Sync Port" {
              }
            }
            n86 = call <instrlib>:"Wait Until Settled.vi"("session in"=w116, "error in"=w117) -> ("session out"=w114:refnum<queue>, "error out"=w115:errorcluster)  [unwired: 12 in]
            n87 = call <instrlib>:"Check Status.vi"("session in"=w114, "error in"=w115) -> ("session out"=w85:refnum<queue>, "error out"=w84:errorcluster)  [unwired: 12 in]
            n88 = call <instrlib>:"LO1 Rx Configure IF Routing.vi"("session in"=w85, "IF signal source"=w111, "error in"=w84) -> ("session out"=w113:refnum<queue>, "error out"=w112:errorcluster)  [unwired: 11 in]
            n89 = call <instrlib>:"LO1 Tx Configure IF Routing.vi"("session in"=w113, "IF signal destination"=w110, "error in"=w112) -> ("error out"=w93:errorcluster)  [unwired: 11 in, 1 out]
            n90 = Index Array(array=w59) -> (element #1=w108:dbl, element #2=w104:dbl)  [unwired: 2 in]
            n91 = Add(x=w107, y=w108) -> (x+y=w106:dbl)
            n92 = Add(x=w102, y=w104) -> (x+y=w103:dbl)
            n93 = Bundle By Name(cluster=w67, "Rx hardware configuration.gain (dB)"=w106, "Tx hardware configuration.gain (dB)"=w103) -> (w105:T3)
          }
          frame True {
            n94 = case shown="\"Transceiver\", Default" w351 {
              tunnel: w352 -> [w371 w383 w390]
              tunnel: [w369 w381 w388] -> w356
              tunnel: w358 -> [w368 w382 w389]
              tunnel: T22 {"Gain Imbalance (linear)"=0.0, "Phase Offset (radians)"=0.0, "Offset "=0.0+0.0i} ("IQ Impairments") -> [w361 w374 w386]
              tunnel: [w359 w372 w385] -> w355
              frame "Receiver" {
                n95 = Unbundle By Name(w371) -> ("rx baseband session.3630 session.VISA resource name"=w370:refnum<visa-resource-name>)
                n96 = call <instrlib>:"Load Baseband IQ Characterization Data.vi"("VISA resource name"=w370, "error in (no error)"=w368) -> ("Characterization Data"=w362:T67, "error out"=w369:errorcluster)  [unwired: 12 in, 4 out]
                n97 = Unbundle By Name(w362) -> ("Imbalance.Gain Imbalance"=w365:dbl, "Imbalance.Phase Imbalance"=w364:dbl, "DC Offset.I DC Offset"=w367:dbl, "DC Offset.Q DC Offset"=w366:dbl)
                n98 = Re/Im To Complex(1:w366, 2:w367) -> (0:w363:cdb)
                n99 = Bundle By Name(cluster=w361, "Gain Imbalance (linear)"=w365, "Phase Offset (radians)"=w364, "Offset"=w363) -> (w360:T22)
                n100 = Build Array(w360) -> (w359:T22[])
              }
              frame "Transmitter" {
                n101 = Unbundle By Name(w383) -> ("tx baseband session.3610 session.VISA resource name"=w384:refnum<visa-resource-name>)
                n102 = call <instrlib>:"Load Baseband IQ Characterization Data.vi"("VISA resource name"=w384, "error in (no error)"=w382) -> ("Characterization Data"=w375:T67, "error out"=w381:errorcluster)  [unwired: 12 in, 4 out]
                n103 = Unbundle By Name(w375) -> ("Imbalance.Gain Imbalance"=w378:dbl, "Imbalance.Phase Imbalance"=w377:dbl, "DC Offset.I DC Offset"=w380:dbl, "DC Offset.Q DC Offset"=w379:dbl)
                n104 = Re/Im To Complex(1:w379, 2:w380) -> (0:w376:cdb)
                n105 = Bundle By Name(cluster=w374, "Gain Imbalance (linear)"=w378, "Phase Offset (radians)"=w377, "Offset"=w376) -> (w373:T22)
                n106 = Build Array(w373) -> (w372:T22[])
              }
              frame "Transceiver", Default {
                n107 = Unbundle By Name(w390) -> ("rx baseband session.3630 session.VISA resource name"=w392:refnum<visa-resource-name>, "tx baseband session.3610 session.VISA resource name"=w391:refnum<visa-resource-name>)
                n108 = Build Array(w392, w391) -> (w387:refnum<visa-resource-name>[])
                n109 = for {
                  shift-right: [w402] -> w388
                  shift-left: w389 -> [w403]
                  tunnel: w387 -> [w401] mode=indexing
                  tunnel: w386 -> [w397]
                  tunnel: [w393] -> w385 mode=indexing
                  n110 = call <instrlib>:"Load Baseband IQ Characterization Data.vi"("VISA resource name"=w401, "error in (no error)"=w403) -> ("Characterization Data"=w400:T67, "error out"=w402:errorcluster)  [unwired: 12 in, 4 out]
                  n111 = Unbundle By Name(w400) -> ("Imbalance.Gain Imbalance"=w396:dbl, "Imbalance.Phase Imbalance"=w395:dbl, "DC Offset.I DC Offset"=w399:dbl, "DC Offset.Q DC Offset"=w398:dbl)
                  n112 = Re/Im To Complex(1:w398, 2:w399) -> (0:w394:cdb)
                  n113 = Bundle By Name(cluster=w397, "Gain Imbalance (linear)"=w396, "Phase Offset (radians)"=w395, "Offset"=w394) -> (w393:T22)
                }
              }
            }
            n114 = call "IQ Impairments impl.vi"("session in"=w352, "direction"=w351, "device configuration"=w350, "IQ Impairments"=w355, "error in (no error)"=w356) -> ("session out"=w353:T6, "error out"=w354:errorcluster)  [unwired: 5 in, 4 out]
          }
        }
      }
    }
    frame Error {
    }
  }
  "error out" <- w7
  "coerced device configuration [channel]" <- w6
  "session out" <- w5
